vi "Read FXP.vi"(7 "FXP Configuration":T1, 8 "error in":errorcluster, 9 "RegisterOffset":u32, 10 "register name":string, 11 "session in":u32) -> (0 "error out":errorcluster, 2 "DBL Value":dbl, 3 "session out":u32)   [LabVIEW 2024, in "FPGA Register IO.lvlib"]
uses:
  FPGA Register IO.lvlib
  TypeDefs/FXP Configuration.ctl
  <vilib>/fxp/LVFixedPointRepBitsTypeDef.ctl
  <vilib>/fxp/LVFixedPointRepRangeTypeDef.ctl
  Error Handling/Error 6003.vi
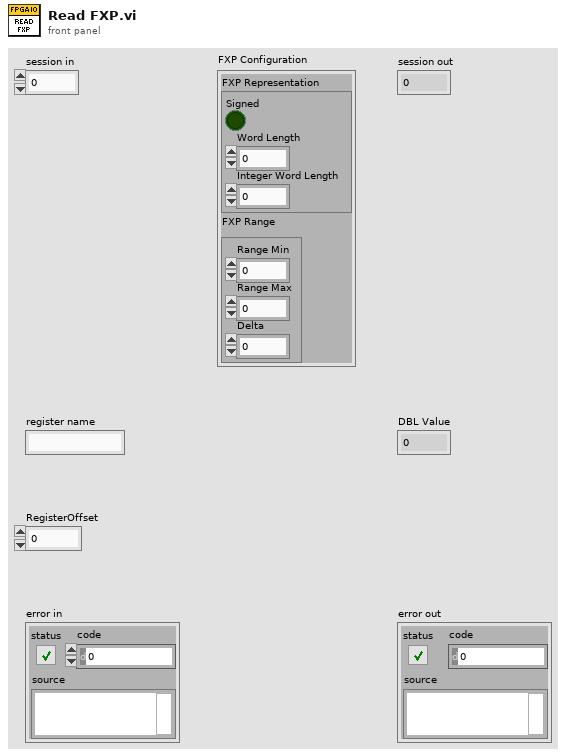
[diagram p1: front panel]
types:
  T1 = typedef "FPGA Register IO.lvlib/FXP Configuration.ctl" = cluster{"FXP Representation":T2, "FXP Range":T3}
  T2 = typedef "LVFixedPointRepBitsTypeDef.ctl" = cluster{"Signed":bool, "Word Length":u32, "Integer Word Length":i32}
  T3 = typedef "LVFixedPointRepRangeTypeDef.ctl" = cluster{"Range Min":dbl, "Range Max":dbl, "Delta":dbl}
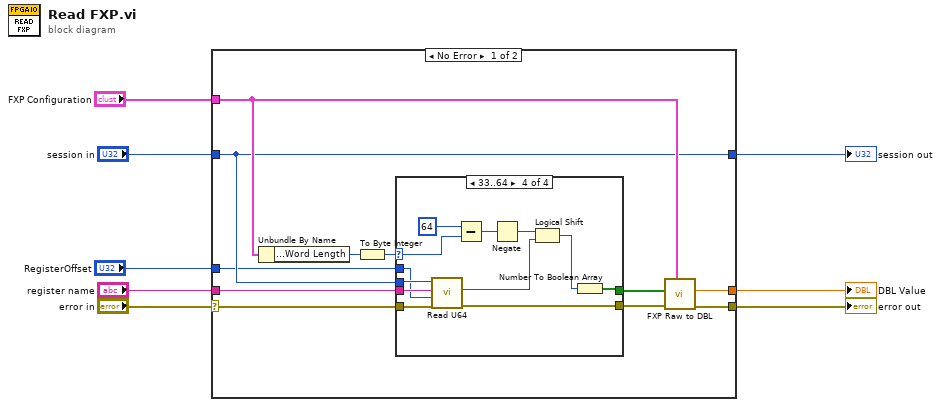
[diagram p0: block diagram]
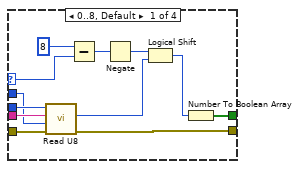
[diagram p2: hidden frame]
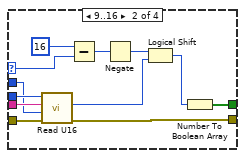
[diagram p3: hidden frame]
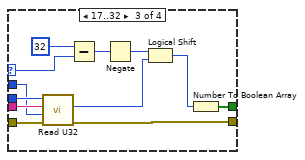
[diagram p4: hidden frame]
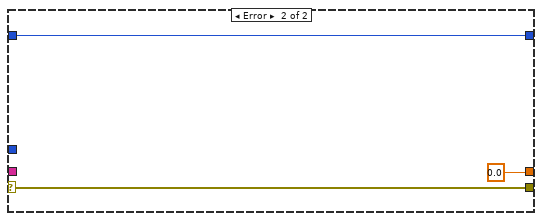
[diagram p5: hidden frame]
diagram:
  n1 = case shown="No Error" "error in" {
    selector: "error in" -> [w12 w70]
    tunnel: "session in" -> [w14 w69]
    tunnel: [w19 w70] -> w8
    tunnel: "register name" -> [w17 _]
    tunnel: [w14 w69] -> w7
    tunnel: [w18 0.0 ("DBL Value")] -> w6
    tunnel: "FXP Configuration" -> [w15 _]
    tunnel: "RegisterOffset" -> [w9 _]
    frame No Error {
      n2 = Unbundle By Name(w15) -> ("FXP Representation.Word Length"=w16:u32)
      n3 = To Byte Integer(number=w16) -> (8bit integer=w10:i8)
      n4 = case shown="33..64" w10 {
        selector: w10 -> [w23 w35 w47 w59]
        tunnel: w17 -> [w30 w41 w53 w65]
        tunnel: [w31 w39 w51 w64] -> w11
        tunnel: w14 -> [w29 w42 w54 w66]
        tunnel: [w28 w40 w52 w63] -> w13
        tunnel: w12 -> [w27 w43 w55 w67]
        tunnel: w9 -> [w20 w32 w44 w56]
        frame 0..8, Default {
          n5 = call "Read U8.vi"("error in"=w27, "RegisterOffset"=w20, "register name"=w30, "session in"=w29) -> ("error out"=w28:errorcluster, "value out"=w22:u8)  [unwired: 5 in, 1 out]
          n6 = Subtract(x=i8 8 ("y"), y=w23) -> (x-y=w25:i8)
          n7 = Negate(x=w25) -> (-x=w24:i8)
          n8 = Logical Shift(y=w24, x=w22) -> (x << y=w21:u8)
          n9 = Number To Boolean Array(number=w21) -> (Boolean array=w31:bool[])
        }
        frame 9..16 {
          n10 = call "Read U16.vi"("error in"=w43, "RegisterOffset"=w32, "register name"=w41, "session in"=w42) -> ("error out"=w40:errorcluster, "value out"=w34:u16)  [unwired: 5 in, 1 out]
          n11 = Subtract(x=i8 16 ("y"), y=w35) -> (x-y=w37:i8)
          n12 = Negate(x=w37) -> (-x=w36:i8)
          n13 = Logical Shift(y=w36, x=w34) -> (x << y=w33:u16)
          n14 = Number To Boolean Array(number=w33) -> (Boolean array=w39:bool[])
        }
        frame 17..32 {
          n15 = call "Read U32.vi"("error in"=w55, "RegisterOffset"=w44, "register name"=w53, "session in"=w54) -> ("error out"=w52:errorcluster, "value out"=w46:u32)  [unwired: 5 in, 1 out]
          n16 = Subtract(x=i8 32 ("y"), y=w47) -> (x-y=w49:i8)
          n17 = Negate(x=w49) -> (-x=w48:i8)
          n18 = Logical Shift(y=w48, x=w46) -> (x << y=w45:u32)
          n19 = Number To Boolean Array(number=w45) -> (Boolean array=w51:bool[])
        }
        frame 33..64 {
          n20 = call "Read U64.vi"("error in"=w67, "RegisterOffset"=w56, "register name"=w65, "session in"=w66) -> ("error out"=w63:errorcluster, "value out"=w58:u64)  [unwired: 5 in, 1 out]
          n21 = Subtract(x=i8 64 ("y"), y=w59) -> (x-y=w61:i8)
          n22 = Negate(x=w61) -> (-x=w60:i8)
          n23 = Logical Shift(y=w60, x=w58) -> (x << y=w57:u64)
          n24 = Number To Boolean Array(number=w57) -> (Boolean array=w64:bool[])
        }
      }
      n25 = call "FXP Raw to DBL.vi"("FXP Configuration"=w15, "error in (no error)"=w13, "Bool Data"=w11) -> ("error out"=w19:errorcluster, "DBL Value"=w18:dbl)  [unwired: 7 in]
    }
    frame Error {
    }
  }
  "error out" <- w8
  "session out" <- w7
  "DBL Value" <- w6
